vi "Search Gain Offset.vi"(8 "Error In":errorcluster, 11 "Input Channel":string) -> (0 "Error Out":errorcluster, 1 "Channel":string, 2 "Offset":dbl, 3 "Gain":dbl, 5 "Name":string)   [LabVIEW 2020]
uses:
  <vilib>/Utility/error.llb/whitespace.ctl
panel:
  # "Y=Gain*x+Offset = (Gain_Offset_Name)Channel or (5.23_3.4_TC1)107"
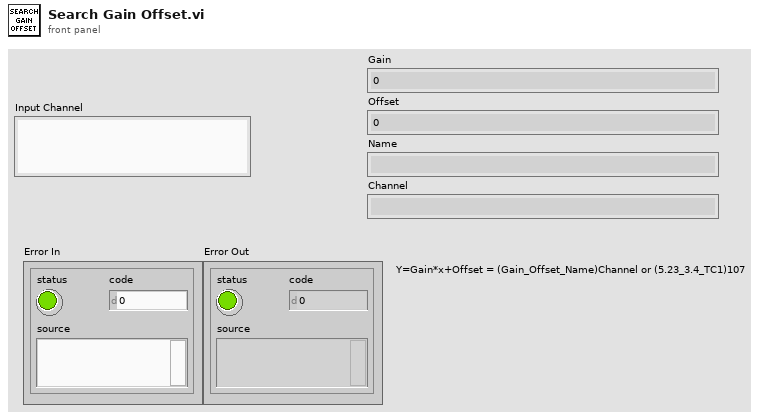
[diagram p1: front panel]
types:
  T1 = typedef "whitespace.ctl" = u16
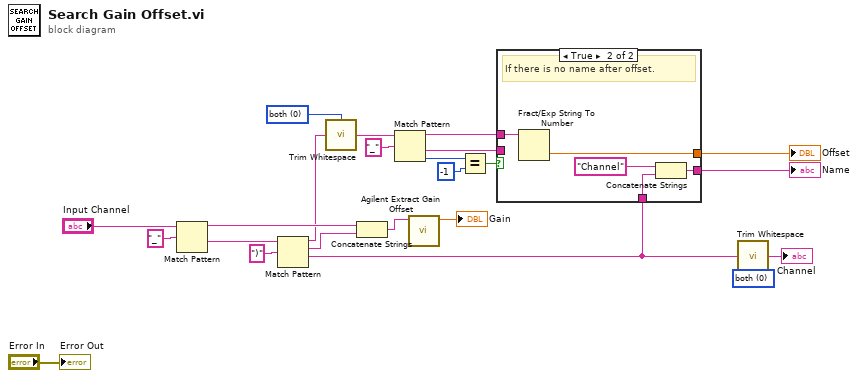
[diagram p0: block diagram]
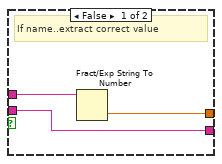
[diagram p2: hidden frame]
diagram:
  w10 = T1 0 items=["both", "start of string", "end of string"] ("location (both)")
  w14 = T1 0 items=["both", "start of string", "end of string"] ("location (both)")
  n1 = Match Pattern(string="Input Channel", regular expression="_") -> (before substring=w19:string, after substring=w20:string)  [unwired: 1 in, 2 out]
  n2 = Match Pattern(string=w20, regular expression=")") -> (before substring=w11:string, match substring=w9:string, after substring=w16:string)  [unwired: 1 in, 1 out]
  n3 = call <vilib>:"Trim Whitespace.vi"("string"=w11, "location (both)"=w10) -> ("trimmed string"=w6:string)
  n4 = Concatenate Strings(w19, w9) -> (w8:string)
  n5 = Match Pattern(string=w6, regular expression="_") -> (before substring=w2:string, after substring=w1:string, offset past match=w5:i32)  [unwired: 1 in, 1 out]
  n6 = call "Agilent Extract Gain Offset.vi"("Gain/Offset"=w8) -> ("Gain/Offset out"=→"Gain":dbl)  [unwired: 9 in, 1 out]
  n7 = Equal?(x=w5, y=-1) -> (x = y?=w3:bool)
  n8 = case shown="True" w3 {
    tunnel: [w26 w31] -> w17
    tunnel: w2 -> [w25 w30]
    tunnel: w1 -> [w24 _]
    tunnel: [w24 w29] -> w13
    tunnel: w16 -> [_ w27]
    frame False {
      # "If name..extract correct value"
      n9 = Fract/Exp String To Number(string=w25) -> (number=w26:dbl)  [unwired: 3 in, 1 out]
    }
    frame True {
      # "If there is no name after offset."
      n10 = Fract/Exp String To Number(string=w30) -> (number=w31:dbl)  [unwired: 3 in, 1 out]
      n11 = Concatenate Strings("Channel" ("string"), w27) -> (w29:string)
    }
  }
  "Offset" <- w17
  "Name" <- w13
  n12 = call <vilib>:"Trim Whitespace.vi"("string"=w16, "location (both)"=w14) -> ("trimmed string"=→"Channel":string)
  "Error Out" <- "Error In"
